vi "读取Distance.vi"(8 "error in (no error)":errorcluster caption="错误输入（无错误）", 11 "Navigation输入":refnum<class "Navigation.lvclass">) -> (0 "error out":errorcluster caption="错误输出", 2 "Distance":dbl, 3 "Navigation输出":refnum<class "Navigation.lvclass">)   [LabVIEW 2018, in "Navigation.lvclass"]
uses:
  Navigation.lvclass
  Navigation.lvclass/Navigation.ctl
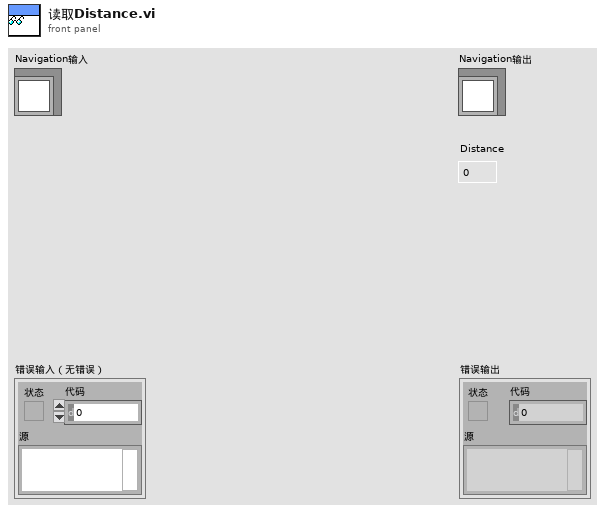
[diagram p1: front panel]
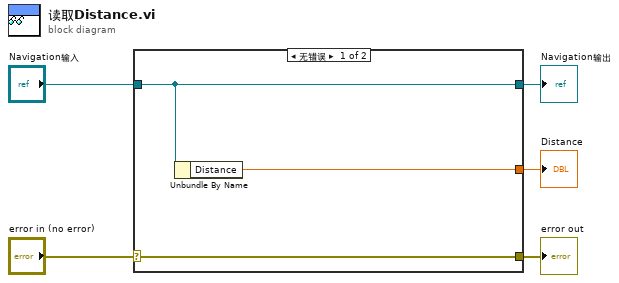
[diagram p0: block diagram]
diagram:
  n1 = case shown="无错误" "error in (no error)" {
    selector: "error in (no error)" -> [w8 w9]
    tunnel: [w8 w9] -> w4
    tunnel: [w7 w10] -> w2
    tunnel: "Navigation输入" -> [w7 w10]
    tunnel: [w6 _] -> w1
    frame No Error {
      n2 = Unbundle By Name(w7) -> ("Distance"=w6:dbl)
    }
    frame Error {
    }
  }
  "error out" <- w4
  "Navigation输出" <- w2
  "Distance" <- w1
